vi "Write Integer Data.vi"(8 "error in (no error)":errorcluster, 10 "Integer Data":T1[](array[typedef]) {"Bit Mask" format="%x"; "Factory Comms Address" format="%x"; "Modbus Address" format="%x"}, 11 "heater_parent in":refnum<class "heater_parent.lvclass">) -> (0 "error out":errorcluster, 3 "heater_parent out":refnum<class "heater_parent.lvclass">)   [LabVIEW 2020, in "polar_bear_plus_drivers.lvlib" / "heater_parent.lvclass"]
uses:
  <instrlib>/RxnRover/Driver Polar Bear Plus/heater_parent/heater_parent.lvclass
  <instrlib>/Eurotherm nanodac/Public/custom controls/Parameter Info.ctl
  <instrlib>/RxnRover/Driver Polar Bear Plus/heater_parent/heater_parent.lvclass/heater_parent.ctl
  <instrlib>/Eurotherm nanodac/Eurotherm nanodac.lvlib
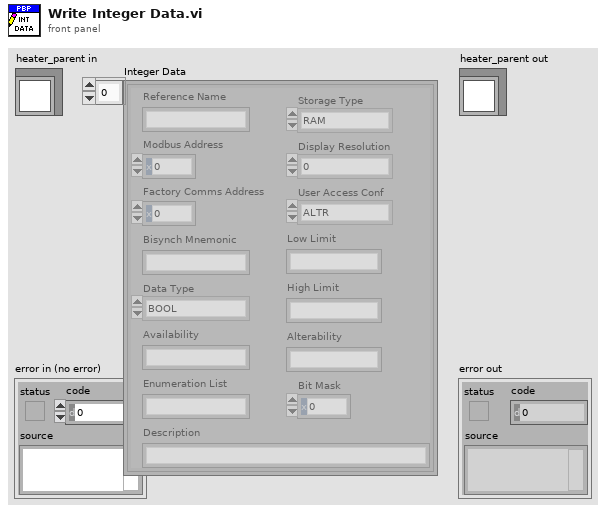
[diagram p1: front panel]
types:
  T1 = typedef "Eurotherm nanodac.lvlib/Parameter Info.ctl" = cluster{"Reference Name":string, "Modbus Address":u16, "Bisynch Mnemonic":string, "Data Type":enum16{"BOOL", "STATE_T", "UINT8", "INT16", "UINT16", "INT32", "UINT32", "TIME_T", "MODBUS_ADDRESS", "FLOAT32", "32BYTES", "EFLOAT32", "ETIME_T", "EINT32", "STRING_T"}, "Availability":string, "Alterability":string, "Low Limit":string, "High Limit":string, "Storage Type":enum16{"RAM", "NON-VOL"}, "Display Resolution":enum16{"0", "1", "2", "PV", "N/A"}, "User Access Conf":enum16{"ALTR", "READ", "HIDE", "N/A"}, "Factory Comms Address":u16, "Enumeration List":string, "Bit Mask":u16, "Description":string}
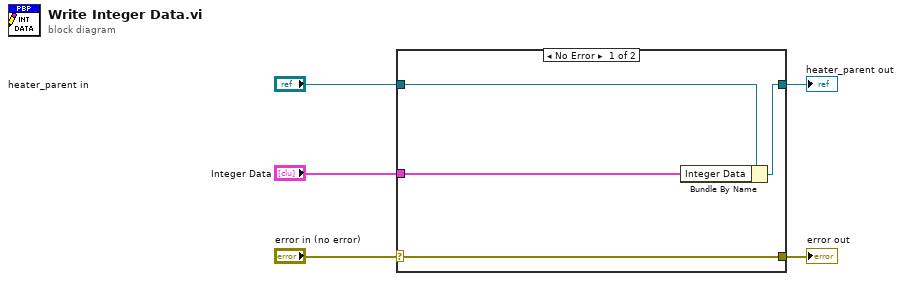
[diagram p0: block diagram]
diagram:
  n1 = case shown="No Error" "error in (no error)" {
    selector: "error in (no error)" -> [w9 w10]
    tunnel: [w9 w10] -> w4
    tunnel: [w7 w11] -> w2
    tunnel: "heater_parent in" -> [w8 w11]
    tunnel: "Integer Data" -> [w6 _]
    frame No Error {
      n2 = Bundle By Name(cluster=w8, "Integer Data"=w6) -> (w7:refnum<class "heater_parent.lvclass">)
    }
    frame Error {
    }
  }
  "error out" <- w4
  "heater_parent out" <- w2
